vi "Deviated_Result_API.vi"(0 "Device DVR In":refnum<data-value>, 11 "Error in":errorcluster) -> (4 "Device DVR Out":refnum<data-value>, 15 "Error Out":errorcluster)   [LabVIEW 2020, in "Device.lvclass"]
doc: "API to calculate Deviated Result"
uses:
  Device.lvclass
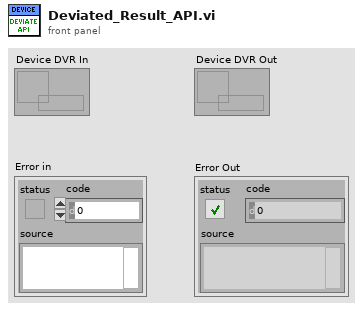
[diagram p1: front panel]
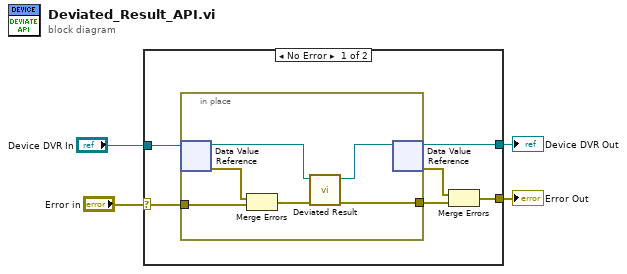
[diagram p0: block diagram]
diagram:
  n1 = case shown="No Error" "Error in" {
    selector: "Error in" -> [w10 w17]
    tunnel: "Device DVR In" -> [w9 w18]
    tunnel: [w7 w18] -> w2
    tunnel: [w6 w17] -> w1
    frame No Error {
      n2 = in-place {
        in-place-border: w10 -> [w16]
        in-place-border: [w11] -> w5
        n3 = in-place-dvr #1(w9) -> (w13:refnum<class "Device.lvclass">, w15:errorcluster)
        n4 = Merge Errors(w15, w16) -> (w14:errorcluster)
        n5 = call-dynamic "Deviated Result.vi"("Error in"=w14, "Device in"=w13) -> ("Error out"=w11:errorcluster, "Device out"=w12:refnum<class "Device.lvclass">)  [unwired: 8 in]
        n6 = in-place-dvr #1(w12) -> (w7:refnum<data-value>, w8:errorcluster)
      }
      n7 = Merge Errors(w8, w5) -> (w6:errorcluster)
    }
    frame Error {
    }
  }
  "Device DVR Out" <- w2
  "Error Out" <- w1
